vi "Start.vi"(8 "error in":errorcluster, 11 "CanHandleIn":T1) -> (0 "error out":errorcluster, 3 "CanHandleOut":T1)   [LabVIEW 2011, in "Konvolucio MCAN120803.lvlib"]
uses:
  <instrlib>/Konvolucio MCAN120803/Konvolucio MCAN120803.lvlib
  <instrlib>/Konvolucio MCAN120803/Types/CanHandleType.ctl
  C:/Program Files/National Instruments/LabVIEW 2011/instr.lib/Konvolucio MCAN120803/Private/Konvolucio.MCAN120803.API.dll
  Private/Konvolucio.MCAN120803.API.dll
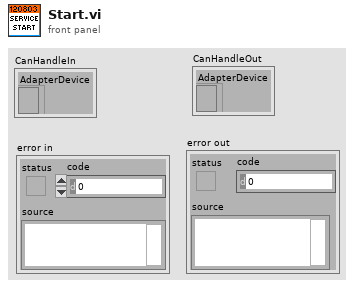
[diagram p1: front panel]
types:
  T1 = typedef "Konvolucio MCAN120803.lvlib/CanHandleType.ctl" = cluster{"AdapterDevice":refnum<k24>}
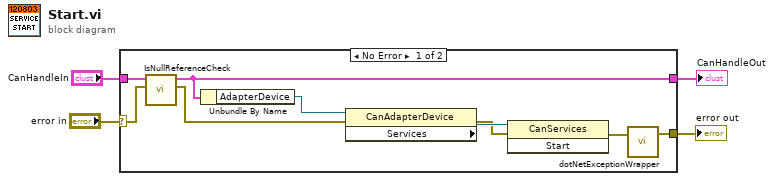
[diagram p0: block diagram]
diagram:
  n1 = case shown="No Error" "error in" {
    selector: "error in" -> [w6 w15]
    tunnel: [w11 w15] -> w4
    tunnel: "CanHandleIn" -> [w7 w14]
    tunnel: [w8 w14] -> w1
    frame No Error {
      n2 = call <instrlib>:"IsNullReferenceCheck.vi"("error in"=w6, "MCanHandleIn"=w7) -> ("error out"=w5:errorcluster, "MCanHandleOut"=w8:T1)  [unwired: 5 in]
      n3 = Unbundle By Name(w8) -> ("AdapterDevice"=w9:refnum<k24>)
      n4 = property class="CanAdapterDevice"(reference=w9, error in=w5) -> (error out=w12:errorcluster, "Services"=w13:refnum<k24>)  [unwired: 1 out]
      n5 = invoke class="CanServices" method="Start"(reference=w13, error in=w12) -> (error out=w10:errorcluster)  [unwired: 1 in, 2 out]
      n6 = call <instrlib>:"dotNetExceptionWrapper.vi"("error in"=w10) -> ("error out"=w11:errorcluster)  [unwired: 2 in]
    }
    frame Error {
    }
  }
  "error out" <- w4
  "CanHandleOut" <- w1
